vi "Set ObjData.vi"(8 "error in (no error)":errorcluster, 10 "Obj Data":T1, 11 "LogEngine":refnum<class "LogEngine.lvclass">) -> (0 "error out":errorcluster, 3 "LogEngine out":refnum<class "LogEngine.lvclass">)   [LabVIEW 2022 SP3, in "LogEngine.lvclass"]
doc: "Developed by Kevin Thompson\nkevin@thompsonengineering.net\n\nCopyright 2018-2020\nThompson Engineering, LLC"
uses:
  LogEngine.lvclass
  LogEngine.lvclass/LogEngine.ctl
  Data Types/TD Logger State--enum.ctl
  Data Types/TD Logger State Data--cluster.ctl
  Data Types/TD LogEngine Settings--cluster.ctl
  DataTypes/SessionSettings--cluster.ctl
  Data Types/LogHeaderData--cluster.ctl
  Data Types/TD Obj Data_LogEngine.ctl
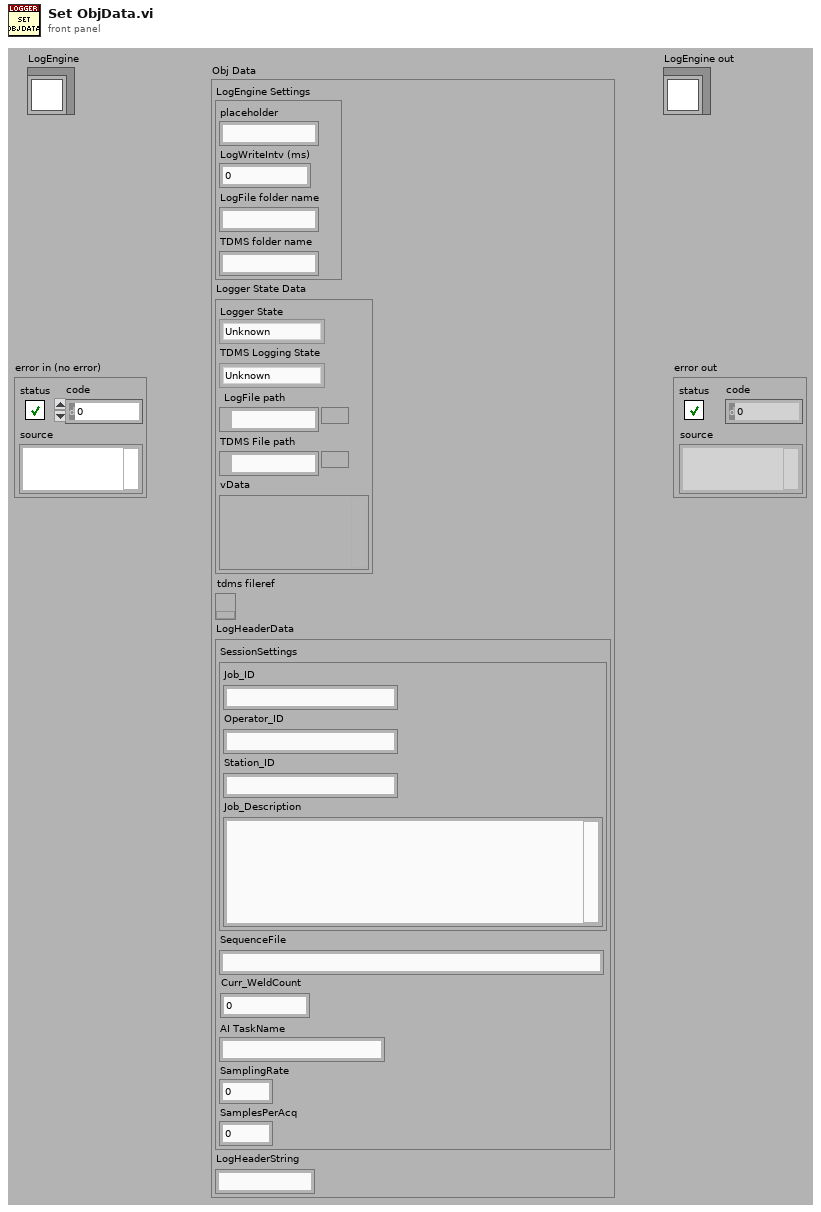
[diagram p1: front panel]
types:
  T1 = typedef "LogEngine.lvclass/TD Obj Data_LogEngine.ctl" = cluster{"LogEngine Settings":T2, "Logger State Data":T3, "tdms fileref":refnum<k34>, "LogHeaderData":T5, "LogHeaderString":string}
  T2 = typedef "LogEngine.lvclass/TD LogEngine Settings--cluster.ctl" = cluster{"placeholder":string, "LogWriteIntv (ms)":u32, "LogFile folder name":string, "TDMS folder name":string}
  T3 = typedef "LogEngine.lvclass/TD Logger State Data--cluster.ctl" = cluster{"Logger State":T4, "TDMS Logging State":T4, "LogFile path":path, "TDMS File path":path, "vData":variant}
  T4 = typedef "LogEngine.lvclass/TD Logger State--enum.ctl" = enum16{"Unknown", "Logging", "NotLogging", "Error"}
  T5 = typedef "LogEngine.lvclass/LogHeaderData--cluster.ctl" = cluster{"SessionSettings":T6, "SequenceFile":string, "Curr_WeldCount":i32, "AI TaskName":string, "SamplingRate":dbl, "SamplesPerAcq":i32}
  T6 = typedef "SessionSettings--cluster.ctl" = cluster{"Job_ID":string, "Operator_ID":string, "Station_ID":string, "Job_Description":string}
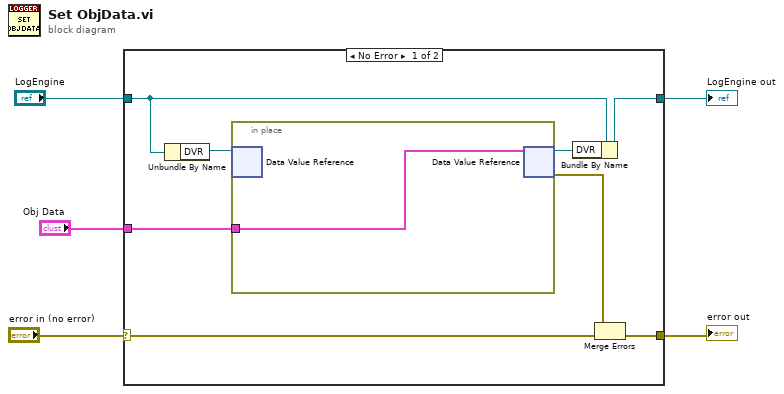
[diagram p0: block diagram]
diagram:
  n1 = case shown="No Error" "error in (no error)" {
    selector: "error in (no error)" -> [w13 w16]
    tunnel: [w8 w16] -> w4
    tunnel: "LogEngine" -> [w11 w15]
    tunnel: [w10 w15] -> w2
    tunnel: "Obj Data" -> [w6 _]
    frame No Error {
      n2 = Unbundle By Name(w11) -> ("DVR"=w12:refnum<data-value>)
      n3 = in-place {
        in-place-border: w6 -> [w14]
        n4 = in-place-dvr #1(w12) -> ()  [unwired: 2 out]
        n5 = in-place-dvr #1(w14) -> (w9:refnum<data-value>, w7:errorcluster)
      }
      n6 = Bundle By Name(cluster=w11, "DVR"=w9) -> (w10:refnum<class "LogEngine.lvclass">)
      n7 = Merge Errors(w7, w13) -> (w8:errorcluster)
    }
    frame Error {
    }
  }
  "error out" <- w4
  "LogEngine out" <- w2
